vi "_CSMObj-Append Chain Node.vi"(7 "Allowed Messages (Empty For All)":string[](array[string]), 8 "Error In":errorcluster caption="error in (no error)", 10 "Requested Name":string, 11 "CSMObj In":T1={"info"={"Module Name"="", "Requested Name"="", "Group Name"="", "Mode"=enum."Stand Alone", "Allowed Messages"=[]}, "Refs"={"WatchDogQ"=refnum, "CSMDataDVR"=refnum, "Queue"={"HPriorityQ"=refnum, "LowPriorityQ"=refnum}, "GroupDataDVR"=refnum, "TagMap"=refnum, "ExitEvent"=refnum, "NewStateEvent"=refnum, "StatusEvent"=refnum, "InterruptEvent"=refnum}}) -> (0 "error out":errorcluster, 2 "Output Cluster (Dup)":T1={"info"={"Module Name"="", "Requested Name"="", "Group Name"="", "Mode"=enum."Stand Alone", "Allowed Messages"=[]}, "Refs"={"WatchDogQ"=refnum, "CSMDataDVR"=refnum, "Queue"={"HPriorityQ"=refnum, "LowPriorityQ"=refnum}, "GroupDataDVR"=refnum, "TagMap"=refnum, "ExitEvent"=refnum, "NewStateEvent"=refnum, "StatusEvent"=refnum, "InterruptEvent"=refnum}}, 3 "CSMObj Out":T1={"info"={"Module Name"="", "Requested Name"="", "Group Name"="", "Mode"=enum."Stand Alone", "Allowed Messages"=[]}, "Refs"={"WatchDogQ"=refnum, "CSMDataDVR"=refnum, "Queue"={"HPriorityQ"=refnum, "LowPriorityQ"=refnum}, "GroupDataDVR"=refnum, "TagMap"=refnum, "ExitEvent"=refnum, "NewStateEvent"=refnum, "StatusEvent"=refnum, "InterruptEvent"=refnum}})   [LabVIEW 2017, in "Communicable State Machine.lvlib"]
uses:
  Communicable State Machine.lvlib
  _CSMObj.ctl
  _CSMObj-Info.ctl
  Typedef/_CSM_MODE.ctl
  _CSMObj-Refs.ctl
  _CSMObj-Data.ctl
  Priority Queue/Priority Queue.ctl
  Typedef/_Cross CSM State Data.ctl
  Typedef/_CSM_MSG_TYPE.ctl
  Typedef/_Cross CSM State Response.ctl
  Typedef/_CSM_Response Source Message.ctl
  Priority Queue/def-Data(LowPRI-Q).ctl
  _CSMObj-ModeData.ctl
  Typedef/_CSM Status Change Event Data.ctl
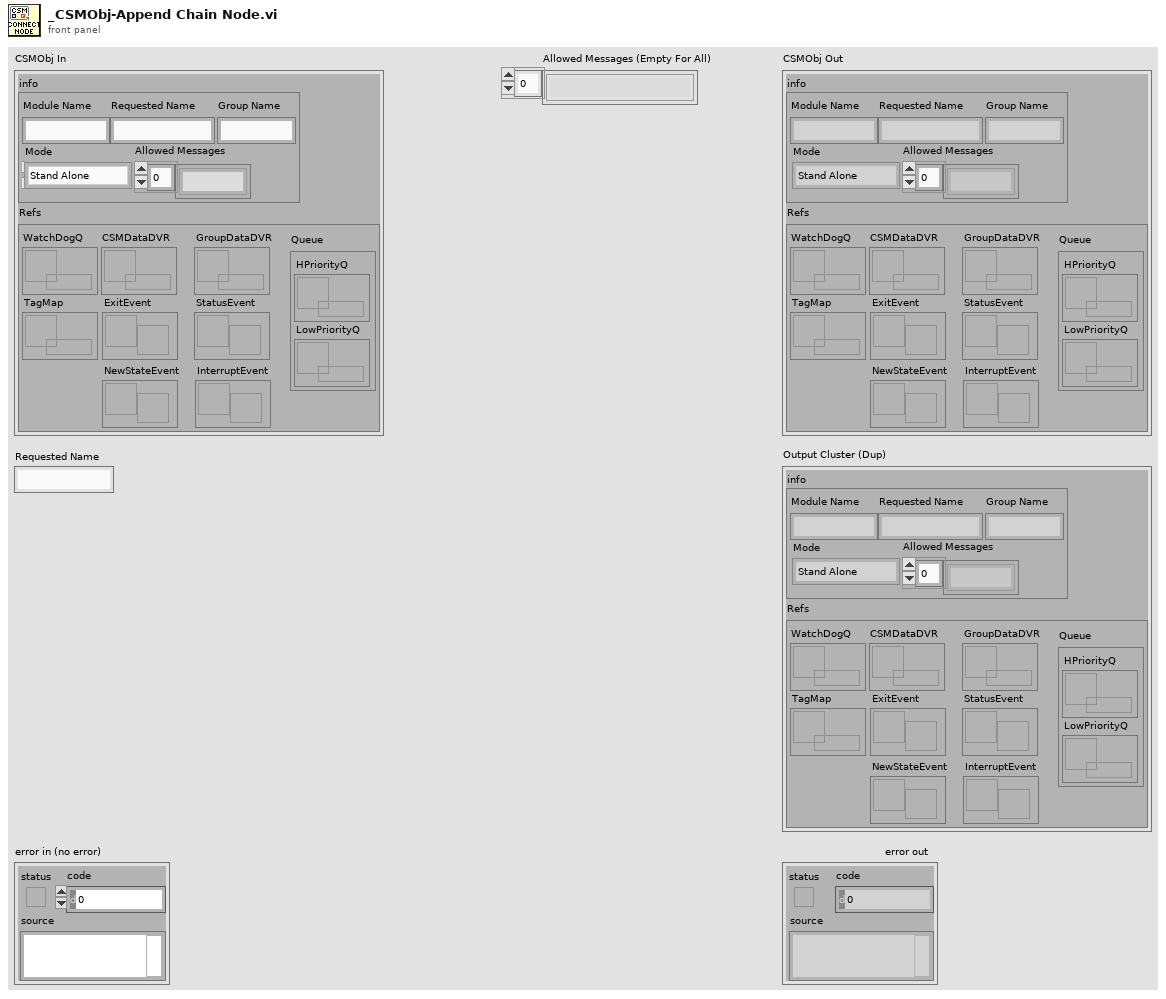
[diagram p1: front panel]
types:
  T1 = typedef "Communicable State Machine.lvlib/_CSMObj.ctl" = cluster{"info":T2, "Refs":T4}
  T2 = typedef "Communicable State Machine.lvlib/_CSMObj-Info.ctl" = cluster{"Module Name":string, "Requested Name":string, "Group Name":string, "Mode":T3, "Allowed Messages":string[]}
  T3 = typedef "Communicable State Machine.lvlib/_CSM_MODE.ctl" = enum16{"Not Exist", "Stand Alone", "CSM", "Worker", "Worker Agent", "Chain Node", "Chain"}
  T4 = typedef "Communicable State Machine.lvlib/_CSMObj-Refs.ctl" = cluster{"WatchDogQ":refnum<queue>, "CSMDataDVR":refnum<data-value>, "Queue":T5, "GroupDataDVR":refnum<data-value>, "TagMap":refnum<data-value>, "ExitEvent":refnum<user-event>, "NewStateEvent":refnum<user-event>, "StatusEvent":refnum<user-event>, "InterruptEvent":refnum<user-event>}
  T5 = typedef "Communicable State Machine.lvlib/Priority Queue.ctl" = cluster{"HPriorityQ":refnum<queue>, "LowPriorityQ":refnum<queue>}
  T6 = typedef "Communicable State Machine.lvlib/_CSMObj-Data.ctl" = cluster{"RemoteMessge?":bool, "error":errorcluster, "Return State":string, "Initialized":enum16{"Initializing", "Ready", "Exiting"}, "InternalRegistryRules":string[]}
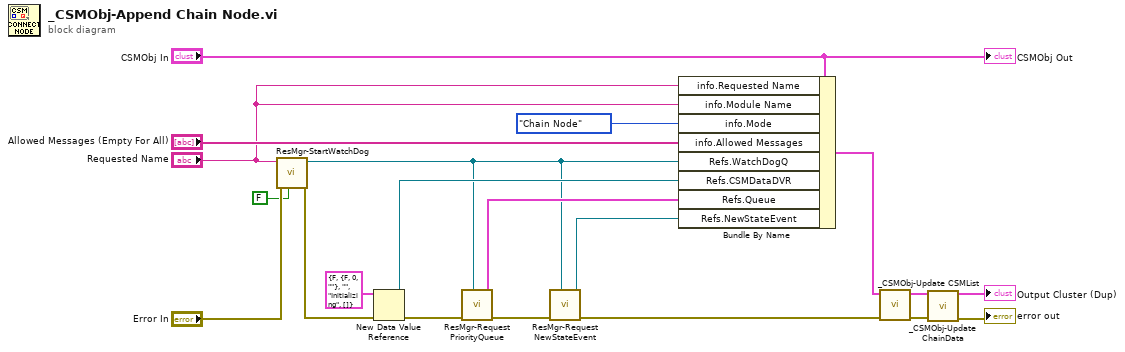
[diagram p0: block diagram]
diagram:
  n1 = call "ResMgr-StartWatchDog.vi"("Force?"=FALSE, "error in (no error)"="Error In", "ModuleName"="Requested Name") -> ("error out"=w12:errorcluster, "WatchDogQ"=w4:refnum<queue>)  [unwired: 7 in]
  n2 = New Data Value Reference(data value=T6 {"RemoteMessge?"=FALSE, "error"={"status"=FALSE, "code"=0, "source"=""}, "Return State"="", "Initialized"=enum."Initializing", "InternalRegistryRules"=[]} ("CSMObj-Data"), error in=w12) -> (data value reference=w19:refnum<data-value>, error out=w11:errorcluster)
  n3 = call "ResMgr-Request PriorityQueue.vi"("WatchDogQ"=w4, "Error In"=w11) -> ("error out"=w3:errorcluster, "Priority Queue"=w10:T5)  [unwired: 8 in]
  n4 = call "ResMgr-Request NewStateEvent.vi"("WatchDogQ"=w4, "Error In"=w3) -> ("error out"=w2:errorcluster, "User Event Out"=w5:refnum<user-event>)  [unwired: 8 in]
  n5 = Bundle By Name(cluster="CSMObj In", "info.Requested Name"="Requested Name", "info.Module Name"="Requested Name", "info.Mode"=_CSM_MODE."Chain Node", "info.Allowed Messages"="Allowed Messages (Empty For All)", "Refs.WatchDogQ"=w4, "Refs.CSMDataDVR"=w19, "Refs.Queue"=w10, "Refs.NewStateEvent"=w5) -> (w15:T1)
  n6 = call "_CSMObj-Update CSMList.vi"("Error In"=w2, "CSMObj In"=w15) -> ("error out"=w16:errorcluster, "CSMObj Out"=w17:T1)  [unwired: 8 in]
  n7 = call "_CSMObj-Update ChainData.vi"("Error In"=w16, "CSMObj In"=w17) -> ("error out"=→"error out":errorcluster, "CSMObj Out"=→"Output Cluster (Dup)":T1)  [unwired: 8 in]
  "CSMObj Out" <- "CSMObj In"
